vi "List Package BuildSpec Version.vi"(8 "error in (no error)":errorcluster, 10 "package buildspec ref in":refnum<vi>, 11 "project ref in":refnum<vi>) -> (0 "error out":errorcluster, 1 "Build Specification Version":T1, 2 "package buildspec ref out":refnum<vi>, 3 "project ref out":refnum<vi>)   [LabVIEW 2018, in "NIPKG BuildSpec API.lvlib"]
uses:
  NIPKG BuildSpec API.lvlib
  <vilib>/AppBuilder/AB_API_Simple/Build Specification Version.ctl
  <vilib>/AppBuilder/AB_API_Simple/NI_App_Builder_API.lvlib
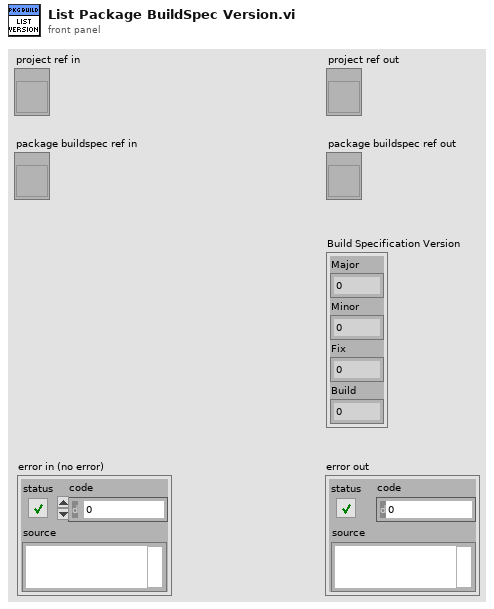
[diagram p1: front panel]
types:
  T1 = typedef "NI_App_Builder_API.lvlib/Build Specification Version.ctl" = cluster{"Major":u16, "Minor":u16, "Fix":u16, "Build":u16}
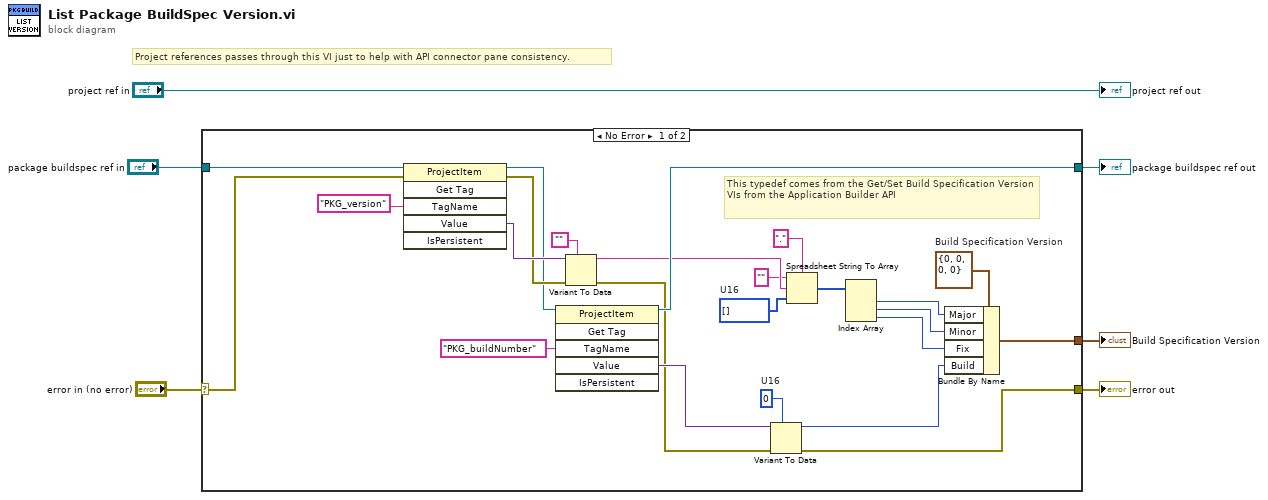
[diagram p0: block diagram]
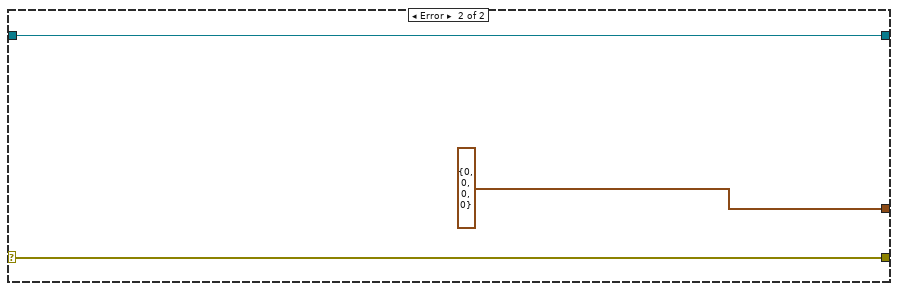
[diagram p2: hidden frame]
diagram:
  # "Project references passes through this VI just to help with API connector pane consistency."
  n1 = case shown="No Error" "error in (no error)" {
    selector: "error in (no error)" -> [w27 w33]
    tunnel: "package buildspec ref in" -> [w28 w31]
    tunnel: [w8 w33] -> w3
    tunnel: [w23 w31] -> w5
    tunnel: [w12 T1 {"Major"=0, "Minor"=0, "Fix"=0, "Build"=0} ("Build Specification Version")] -> w1
    frame No Error {
      w7 = u16 0  # U16
      w17 = T1 {"Major"=0, "Minor"=0, "Fix"=0, "Build"=0}  # Build Specification Version
      w19 = u16[] []  # U16
      # "This typedef comes from the Get/Set Build Specification Version VIs from the Application Builder API"
      n2 = invoke class="ProjectItem" method="Get Tag"(reference=w28, error in=w27, "TagName"="PKG_version" ("Tag Name")) -> (reference out=w24:refnum<vi>, error out=w25:errorcluster, "Value"=w29:variant)  [unwired: 3 in, 3 out]
      n3 = invoke class="ProjectItem" method="Get Tag"(reference=w24, "TagName"="PKG_buildNumber" ("Tag Name")) -> (reference out=w23:refnum<vi>, "Value"=w11:variant)  [unwired: 4 in, 4 out]
      n4 = Variant To Data(error in=w25, type="", Variant=w29) -> (data=w21:string, error out=w9:errorcluster)
      n5 = Variant To Data(error in=w9, type=w7, Variant=w11) -> (data=w10:u16, error out=w8:errorcluster)
      n6 = Spreadsheet String To Array(delimiter (Tab)=".", format string="", spreadsheet string=w21, array type (2D Dbl)=w19) -> (array=w16:u16[])
      n7 = Index Array(array=w16) -> (element #1=w15:u16, element #2=w14:u16, element #3=w13:u16)  [unwired: 3 in]
      n8 = Bundle By Name(cluster=w17, "Major"=w15, "Minor"=w14, "Fix"=w13, "Build"=w10) -> (w12:T1)
    }
    frame Error {
    }
  }
  "package buildspec ref out" <- w5
  "error out" <- w3
  "Build Specification Version" <- w1
  "project ref out" <- "project ref in"
